vi "SelectCurString2DListCtrl.vi"(7 "clicked seq list?":bool, 8 "string":string, 9 "combo in":refnum<vi>, 10 "column index":u16, 11 "list in":refnum<vi>) -> (3 "list out":refnum<vi>)   [LabVIEW 2018, in "Library-Ctrl.lvlib"]
uses:
  Library-Ctrl.lvlib
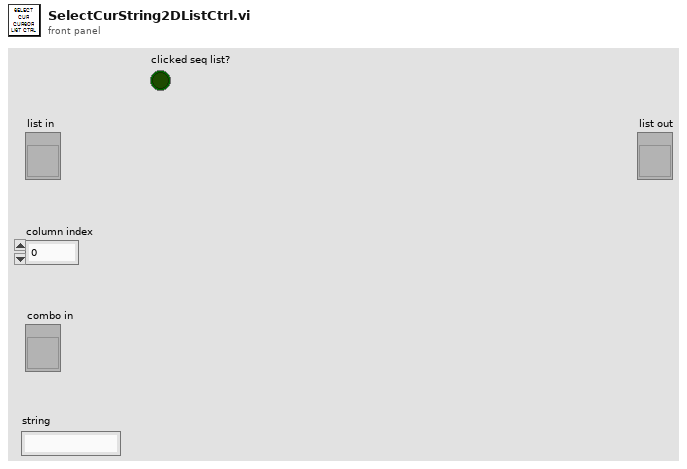
[diagram p1: front panel]
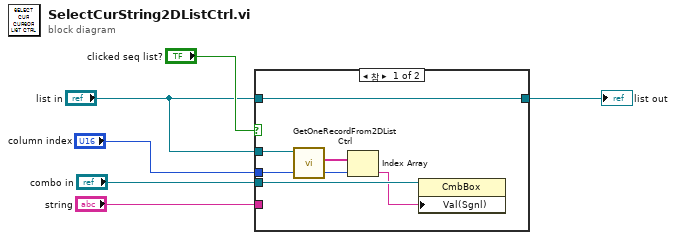
[diagram p0: block diagram]
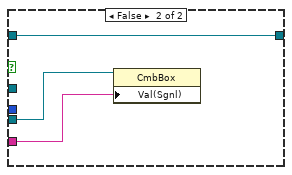
[diagram p2: hidden frame]
diagram:
  n1 = case shown="참" "clicked seq list?" {
    tunnel: "combo in" -> [w10 w15]
    tunnel: "string" -> [_ w14]
    tunnel: "list in" -> [w12 _]
    tunnel: "column index" -> [w8 _]
    tunnel: [w7 w13] -> w2
    tunnel: "list in" -> [w7 w13]
    frame True {
      n2 = call "GetOneRecordFrom2DListCtrl.vi"("testcaselist in"=w12) -> ("one record"=w11:string[])  [unwired: 9 in, 1 out]
      n3 = Index Array(array=w11, index=w8) -> (element=w9:string)
      n4 = property class="CmbBox"(reference=w10, "Val(Sgnl)"=w9) -> ()  [unwired: 1 in, 2 out]
    }
    frame False {
      n5 = property class="CmbBox"(reference=w15, "Val(Sgnl)"=w14) -> ()  [unwired: 1 in, 2 out]
    }
  }
  "list out" <- w2
